vi "Sub_getEigensolution.vi"(10 "MASS":T1, 11 "STIFF":T1) -> (0 "MASS":T1, 1 "STIFF":T1, 2 "Eigenvectors":T1, 3 "Eigenvalues":cdb[](array[numeric]))   [LabVIEW 2019]
uses:
  <vilib>/Analysis/Matrix/Datatypes/RealMatrix.ctl
  <vilib>/Analysis/7linalg.llb/Real Generalized Eigenvalues and Vectors.vi
  <vilib>/Analysis/NI_AALPro.lvlib
  <vilib>/Analysis/Matrix/NI_Matrix.lvlib
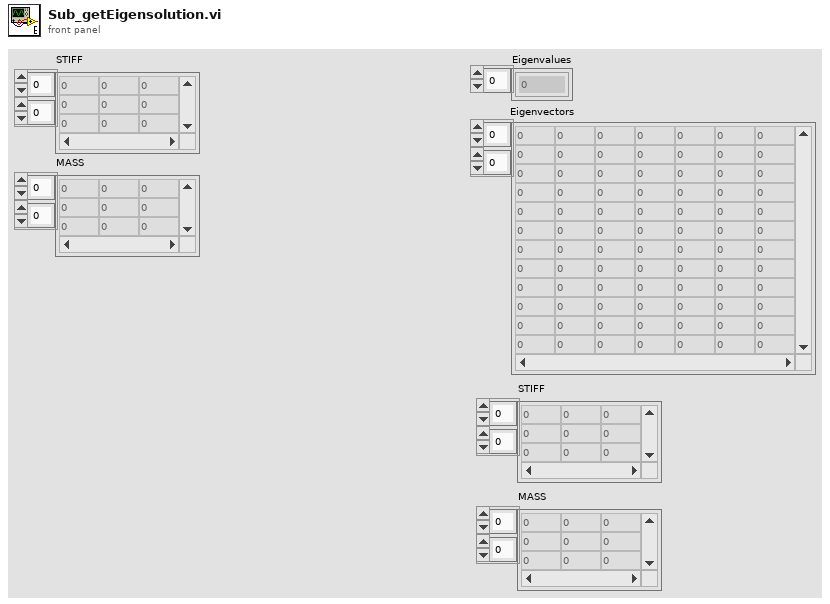
[diagram p1: front panel]
types:
  T1 = typedef "NI_Matrix.lvlib/RealMatrix.ctl" = dbl[][]
  T2 = typedef "NI_Matrix.lvlib/ComplexMatrix.ctl" = cdb[][]
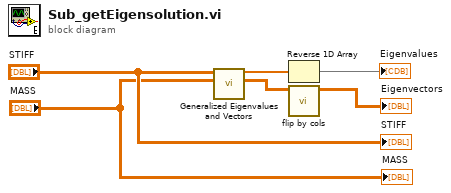
[diagram p0: block diagram]
diagram:
  n1 = call-poly <vilib>:"Generalized Eigenvalues and Vectors.vi"("B"="MASS", "A"="STIFF") -> ("Eigenvectors"=w2:T2, "Eigenvalues"=w4:cdb[])  [unwired: 4 in, 1 out]
  n2 = Reverse 1D Array(array=w4) -> (reversed array=→"Eigenvalues":cdb[])
  n3 = call "flip by cols.vi"("Matrix"=w2) -> ("Flipped by Cols"=→"Eigenvectors":T1)  [unwired: 10 in]
  "MASS" <- "MASS"
  "STIFF" <- "STIFF"
